vi "Main_Dynamic-Window-Approach.vi"() -> ()   [LabVIEW 2019]
uses:
  Ctrl/cmd_common.ctl
panel:
  in  "yaw rate resolution":dbl=0.1
  in  "max delta yaw rate":dbl=40.0
  in  "max yaw rate":dbl=40.0
  in  "config":T1={"max speed"=1.0, "min speed"=-0.5, "max yaw rate"=0.0, "max accel"=0.2, "max delta yaw rate"=0.0, "v resolution"=0.01, "yaw rate resolution"=0.0, "dt"=0.1, "predict time"=3.0, "to goal cost gain"=0.15, "speed cost gain"=1.0, "obstacle cost gain"=1.0, "robot stuck flag cons"=0.001, "robot type"=enum."rectangle", "robot radius"=1.0, "robot width"=0.5, "robot length"=1.2, "obstacles"=[{"x"=-1.0, "y"=-1.0}, {"x"=0.0, "y"=2.0}, {"x"=4.0, "y"=2.0}, {"x"=5.0, "y"=4.0}, {"x"=5.0, "y"=5.0}, {"x"=5.0, "y"=6.0}, {"x"=5.0, "y"=9.0}, {"x"=8.0, "y"=9.0}, {"x"=7.0, "y"=9.0}, {"x"=8.0, "y"=10.0}, {"x"=9.0, "y"=11.0}, {"x"=12.0, "y"=13.0}, {"x"=12.0, "y"=12.0}, {"x"=15.0, "y"=15.0}, {"x"=13.0, "y"=13.0}], "goal pt"={"x"=10, "y"=10}}
  out "Numeric":i32
  in  "stop":bool
  in  "yaw":dbl=8.0 format="%#_13g"
  # "# initial state [x(m), y(m), yaw(rad), v(m/s), omega(rad/s)]"
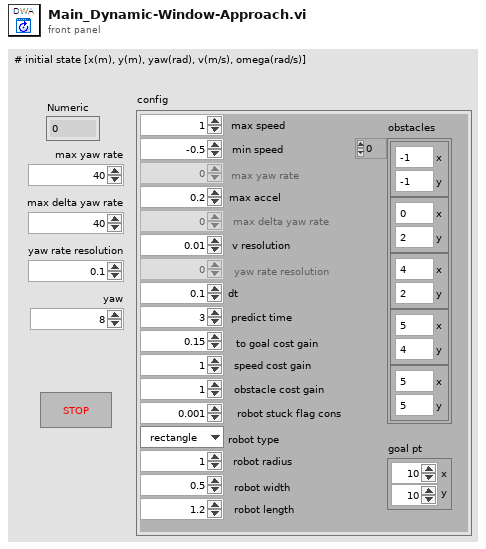
[diagram p1: front panel]
types:
  T1 = cluster{"max speed":dbl, "min speed":dbl, "max yaw rate":dbl, "max accel":dbl, "max delta yaw rate":dbl, "v resolution":dbl, "yaw rate resolution":dbl, "dt":dbl, "predict time":dbl, "to goal cost gain":dbl, "speed cost gain":dbl, "obstacle cost gain":dbl, "robot stuck flag cons":dbl, "robot type":enum16{"circle", "rectangle"}, "robot radius":dbl, "robot width":dbl, "robot length":dbl, "obstacles":cluster{"x":dbl, "y":dbl}[], "goal pt":cluster{"x":i32, "y":i32}}
  T2 = typedef "cmd_common.ctl" = enum16{"read", "write"}
  T3 = cluster{"x":dbl[], "dw":dbl[], "u":cluster{"v":dbl, "y":dbl}, "trajectory":dbl[][], "best trajectory":dbl[][], "best u":cluster{"v":dbl, "y":dbl}}
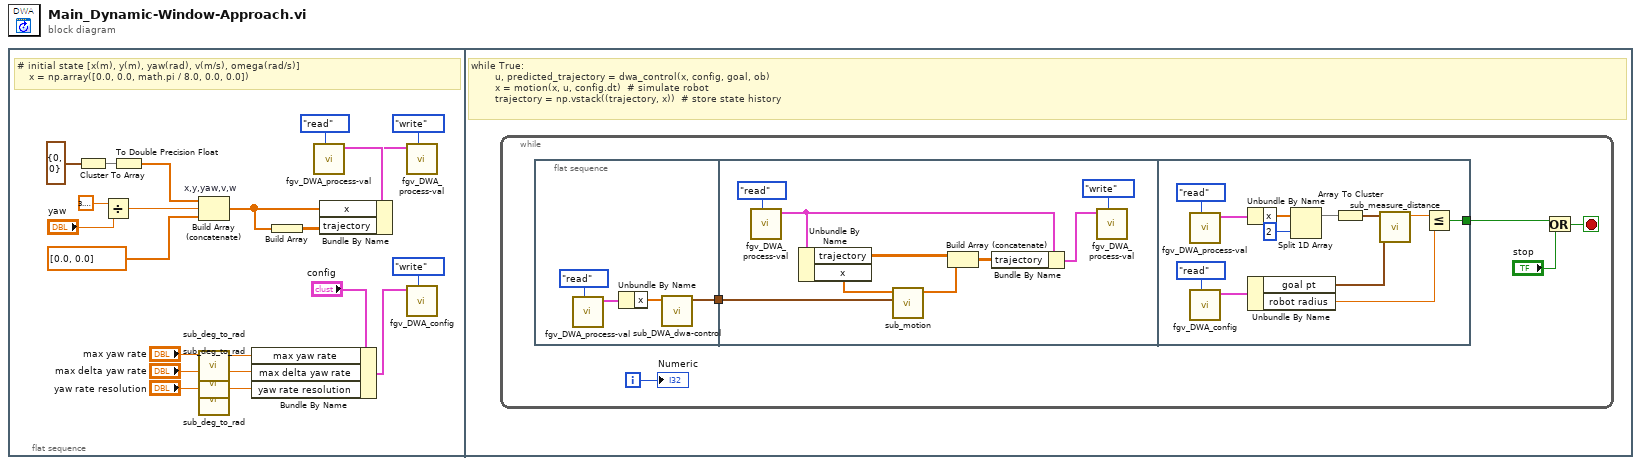
[diagram p0: block diagram]
diagram:
  n1 = flat-sequence {
    frame #0 {
      # "# initial state [x(m), y(m), yaw(rad), v(m/s), omega(rad/s)]\n    x = np.array([0.0, 0.0, math.pi / 8.0, 0.0, 0.0])"
      n2 = Cluster To Array(cluster=cluster{"x":i32, "y":i32} {"x"=0, "y"=0} ("goal pt")) -> (array=w18:i32[])
      n3 = Divide(x=3.141592653589793, y="yaw") -> (x/y=w20:dbl)
      n4 = To Double Precision Float(number=w18) -> (double precision float=w17:dbl[])
      n5 = Build Array (concatenate) "x,y,yaw,v,w"(w17, w20, dbl[] [0.0, 0.0] ("double precision float")) -> (w1:dbl[])
      n6 = call "sub_deg_to_rad.vi"("deg in"="max yaw rate") -> ("rad out"=w3:dbl)  [unwired: 10 in]
      n7 = call "sub_deg_to_rad.vi"("deg in"="max delta yaw rate") -> ("rad out"=w4:dbl)  [unwired: 10 in]
      n8 = call "sub_deg_to_rad.vi"("deg in"="yaw rate resolution") -> ("rad out"=w5:dbl)  [unwired: 10 in]
      n9 = Bundle By Name(cluster="config", "max yaw rate"=w3, "max delta yaw rate"=w4, "yaw rate resolution"=w5) -> (w6:T1)
      n10 = Build Array(w1) -> (w2:dbl[][])
      n11 = call "fgv_DWA_process-val.vi"("cmd"=cmd_common."read") -> ("prcess val out"=w12:T3)  [unwired: 10 in]
      n12 = Bundle By Name(cluster=w12, "x"=w1, "trajectory"=w2) -> (w11:T3)
      n13 = call "fgv_DWA_process-val.vi"("cmd"=cmd_common."write", "prcess val"=w11) -> ()  [unwired: 9 in, 1 out]
      n14 = call "fgv_DWA_config.vi"("cmd"=cmd_common."write", "config"=w6) -> ()  [unwired: 9 in, 1 out]
    }
    frame #1 {
      # "while True:\n        u, predicted_trajectory = dwa_control(x, config, goal, ob)\n        x = motion(x, u, config.dt)  # simulate robot\n        trajectory = np.vstack((trajectory, x))  # store state history"
      n15 = while {
        i -> [w27]
        stop <- w24 stop-if-true
        n16 = flat-sequence {
          tunnel: [w28] -> w23
          tunnel: w23 -> [w33]
          tunnel: [w41] -> w26
          frame #0 {
            n17 = call "fgv_DWA_process-val.vi"("cmd"=cmd_common."read") -> ("prcess val out"=w30:T3)  [unwired: 10 in]
            n18 = Unbundle By Name(w30) -> ("x"=w29:dbl[])
            n19 = call "sub_DWA_dwa-control.vi"("x"=w29) -> ("u"=w28:cluster{"v":dbl, "y":dbl})  [unwired: 9 in, 1 out]
          }
          frame #1 {
            n20 = call "fgv_DWA_process-val.vi"("cmd"=cmd_common."read") -> ("prcess val out"=w38:T3)  [unwired: 10 in]
            n21 = Unbundle By Name(w38) -> ("trajectory"=w40:dbl[][], "x"=w32:dbl[])
            n22 = call "sub_motion.vi"("u"=w33, "x"=w32) -> ("x out"=w34:dbl[])  [unwired: 9 in]
            n23 = Build Array (concatenate)(w40, w34) -> (w39:dbl[][])
            n24 = Bundle By Name(cluster=w38, "trajectory"=w39) -> (w37:T3)
            n25 = call "fgv_DWA_process-val.vi"("cmd"=cmd_common."write", "prcess val"=w37) -> ()  [unwired: 9 in, 1 out]
          }
          frame #2 {
            n26 = call "fgv_DWA_process-val.vi"("cmd"=cmd_common."read") -> ("prcess val out"=w51:T3)  [unwired: 10 in]
            n27 = call "fgv_DWA_config.vi"("cmd"=cmd_common."read") -> ("config out"=w49:T1)  [unwired: 10 in]
            n28 = Unbundle By Name(w51) -> ("x"=w48:dbl[])
            n29 = Unbundle By Name(w49) -> ("goal pt"=w44:cluster{"x":i32, "y":i32}, "robot radius"=w42:dbl)
            n30 = Split 1D Array(array=w48, index=2 ("인덱스")) -> (first subarray=w46:dbl[])  [unwired: 1 out]
            n31 = Array To Cluster(array=w46) -> (cluster=w45:cluster{"[0]":dbl, "[1]":dbl})
            n32 = call "sub_measure_distance.vi"("pt 2"=w44, "pt 1"=w45) -> ("distance"=w43:dbl)  [unwired: 9 in]
            n33 = Less Or Equal?(x=w43, y=w42) -> (x <= y?=w41:bool)
          }
        }
        n34 = Or(x=w26, y="stop") -> (x .or. y?=w24:bool)
        "Numeric" <- w27
      }
    }
  }
